vi "Get Active VI of Active Project.vi"(8 "error in (no error)":errorcluster, 11 "App Ref":refnum<vi>) -> (0 "error out":errorcluster, 3 "Active VI Ref":refnum<vi>)   [LabVIEW 2020, in "MacroAssert.lvlib"]
doc: "Gets the active (or frontmost) VI within <B>App Ref</B> in the situation where App.Kind is Development System."
uses:
  MacroAssert.lvlib
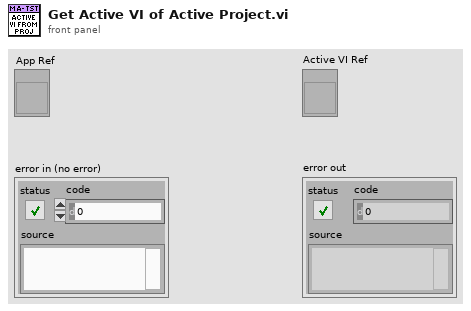
[diagram p1: front panel]
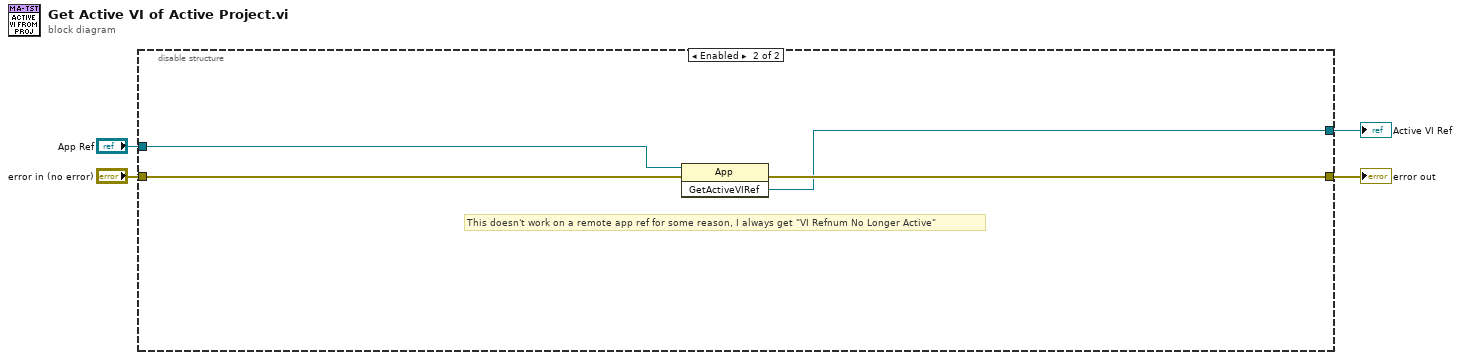
[diagram p0: block diagram]
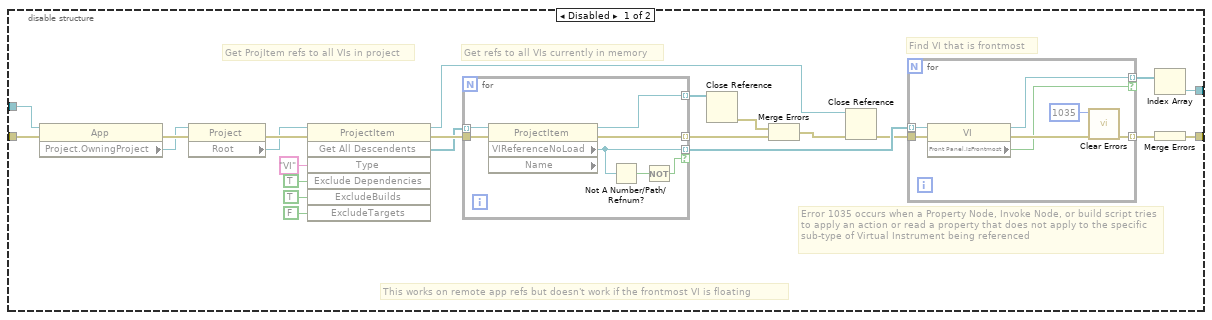
[diagram p2: hidden frame]
diagram:
  n1 = disable-structure shown="Enabled" {
    disable-tunnel: [w27 w43] -> w4
    disable-tunnel: "error in (no error)" -> [w26 w45]
    disable-tunnel: "App Ref" -> [w25 w44]
    disable-tunnel: [w24 w42] -> w1
    frame Disabled {
      # "This works on remote app refs but doesn't work if the frontmost VI is floating"
      # "Error 1035 occurs when a Property Node, Invoke Node, or build script tries to apply an action or read a property that does not apply to the specific sub-type of Virtual Instrument being referenced"
      # "Find VI that is frontmost"
      # "Get ProjItem refs to all VIs in project"
      # "Get refs to all VIs currently in memory"
      n2 = property class="App"(reference=w25, error in=w26) -> (error out=w23:errorcluster, "Project.OwningProject"=w17:refnum<vi>)  [unwired: 1 out]
      n3 = property class="Project"(reference=w17, error in=w23) -> (error out=w22:errorcluster, "Root"=w18:refnum<vi>)  [unwired: 1 out]
      n4 = invoke class="ProjectItem" method="Get All Descendents"(reference=w18, error in=w22, "Type"="VI", "Exclude Dependencies"=TRUE ("ExcludeDependencies"), "ExcludeBuilds"=TRUE, "ExcludeTargets"=FALSE) -> (reference out=w5:refnum<vi>, error out=w21:errorcluster, "All Descendents"=w16:refnum<vi>[])  [unwired: 1 in, 4 out]
      n5 = for {
        tunnel: w16 -> [w39] mode=indexing
        tunnel: [w38] -> w11 mode=indexing
        tunnel: [w37] -> w10 mode=indexing if=w35
        tunnel: w21 -> [w41]
        tunnel: [w40] -> w7 mode=indexing
        n6 = property class="ProjectItem" props=["VIReferenceNoLoad", "Name"](reference=w39, error in=w41) -> (reference out=w38:refnum<vi>, error out=w40:errorcluster, "VIReferenceNoLoad"=w37:refnum<vi>)  [unwired: 1 out]
        n7 = Not A Number/Path/Refnum?(number/path/refnum=w37) -> (NaN/Path/Refnum?=w36:bool)
        n8 = Not(x=w36) -> (.not. x?=w35:bool)
      }
      n9 = Close Reference(reference=w11) -> (error out=w20:errorcluster)  [unwired: 1 in]
      n10 = Merge Errors(w20, w7) -> (w19:errorcluster)
      n11 = Close Reference(reference=w5, error in (no error)=w19) -> (error out=w6:errorcluster)
      n12 = for {
        tunnel: w10 -> [w32] mode=indexing
        tunnel: [w28] -> w9 mode=indexing if=w31
        tunnel: [w30] -> w8 mode=indexing
        tunnel: w6 -> [w33]
        n13 = property class="VI"(reference=w32, error in=w33) -> (reference out=w28:refnum<vi>, error out=w34:errorcluster, "Front Panel.IsFrontmost"=w31:bool)
        n14 = call <vilib>:"Clear Errors.vi"("error in (no error)"=w34, "specific error code to clear (0: all)"=1035) -> ("error out"=w30:errorcluster)  [unwired: 4 in, 1 out]
      }
      n15 = Index Array(array=w9) -> (element=w24:refnum<vi>)  [unwired: 1 in]
      n16 = Merge Errors(w8) -> (w27:errorcluster)
    }
    frame Enabled {
      # "This doesn't work on a remote app ref for some reason, I always get \"VI Refnum No Longer Active\""
      n17 = invoke class="App" method="GetActiveVIRef"(reference=w44, error in=w45) -> (error out=w43:errorcluster, "GetActiveVIRef"=w42:refnum<vi>)  [unwired: 1 in, 1 out]
    }
  }
  "error out" <- w4
  "Active VI Ref" <- w1
